vi "Process Memory Monitor.vi"() -> ()   [LabVIEW 2016]
panel:
  in  "Process Info Tab":enum32{"Page 1", "Page 2"}(tab)
  out "LabVIEW HandleCount":u32
  out "LabVIEW Thread Count":u32
  out "LabVIEW Memory Used (MB)":u64
  out "Sequence Editor Memory (MB)":u64
  out "Sequence Editor  HandleCount":u32
  out "Sequence Editor Thread Count":u32
  out "Process Memory Used (MB)":u64
  out "Process Thread Count":u32
  out "Process HandleCount":u32
  in  "Process Name (optional)":string
  in  "Log File Path":path=path "C:/Users/zhyang/Desktop/log.csv"
  in  "Interval (s)":dbl=3.0
  out "Memory Usage":cluster{"HandleCount":dbl, "HandleCount":dbl}(graph)
  out "error out":errorcluster
  in  "stop":bool
  # "Process Name is optional. If you let the control empty, this VI will monitor the LabVIEW and TestStand memory usage."
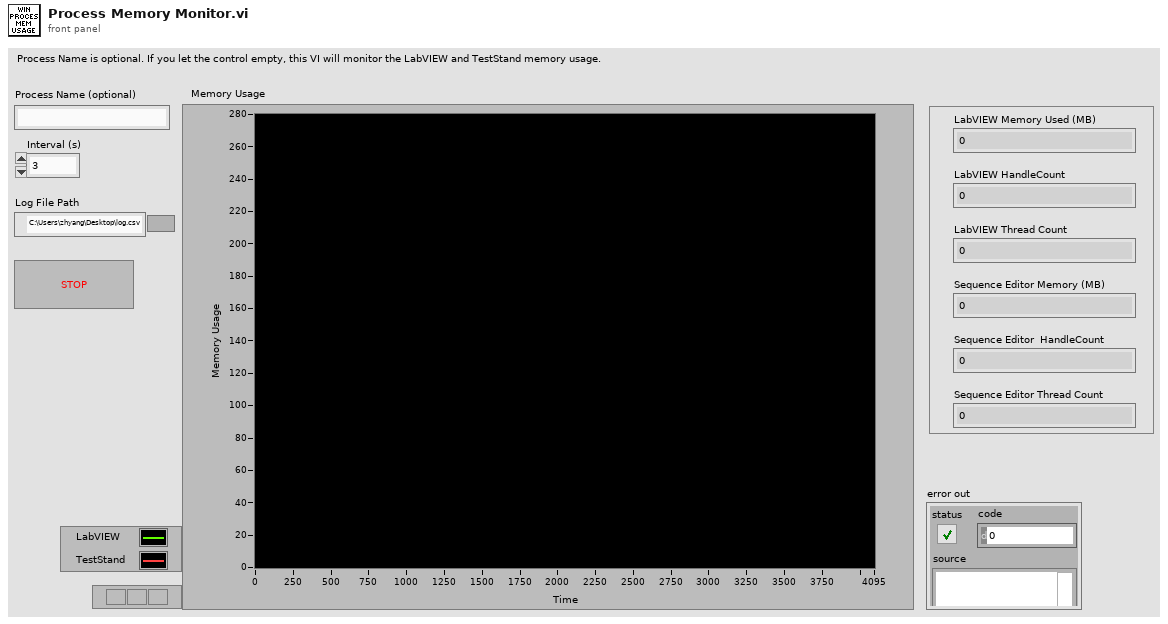
[diagram p1: front panel]
types:
  T1 = cluster{"LabVIEW  Memory Used (MB)":dbl, "Sequence Editor Memory (MB)":dbl}
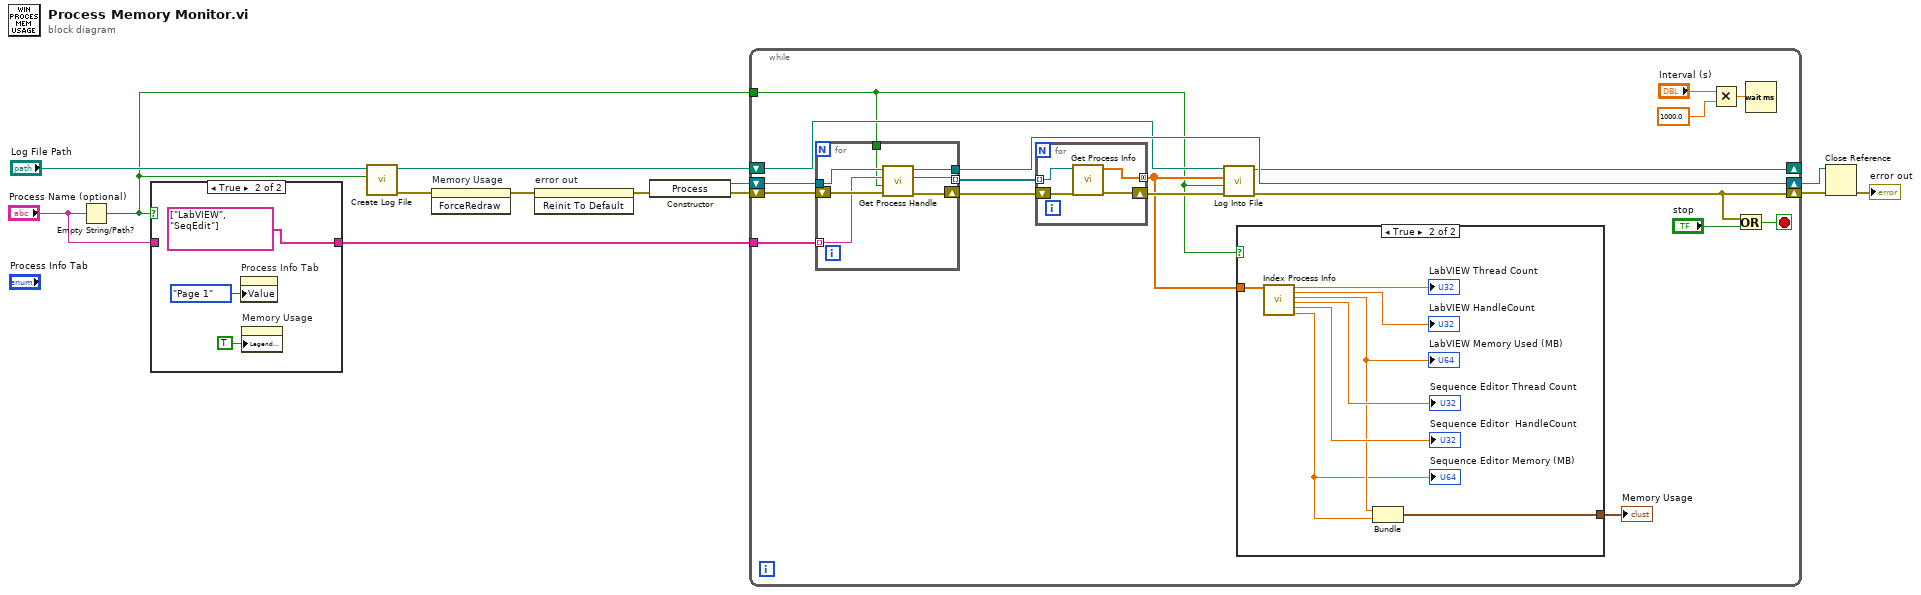
[diagram p0: block diagram]
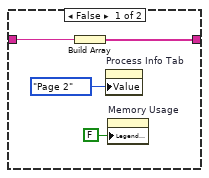
[diagram p2: hidden frame]
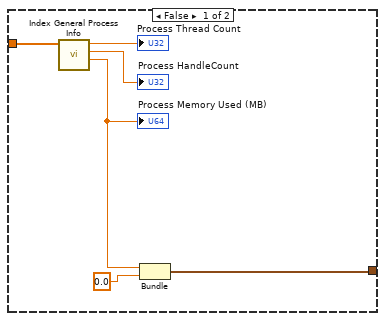
[diagram p3: hidden frame]
diagram:
  n1 = Empty String/Path?(string/path="Process Name (optional)") -> (empty?=w1:bool)
  n2 = case shown="True" w1 {
    tunnel: [w16 string[] ["LabVIEW", "SeqEdit"]] -> w2
    tunnel: "Process Name (optional)" -> [w17 _]
    frame False {
      n3 = Build Array(w17) -> (w16:string[])
      n4 = property on="Process Info Tab" class="TabCtl (strict)"("Value"=enum32{"Page 1", "Page 2"}."Page 2" ("Process Info Tab")) -> ()  [unwired: 2 in, 2 out]
      n5 = property on="Memory Usage" class="WFChart (strict)"("Legend Visible"=FALSE ("Legend:Visible")) -> ()  [unwired: 2 in, 2 out]
    }
    frame True {
      n6 = property on="Process Info Tab" class="TabCtl (strict)"("Value"=enum32{"Page 1", "Page 2"}."Page 1" ("Process Info Tab")) -> ()  [unwired: 2 in, 2 out]
      n7 = property on="Memory Usage" class="WFChart (strict)"("Legend Visible"=TRUE ("Legend:Visible")) -> ()  [unwired: 2 in, 2 out]
    }
  }
  n8 = call "Create Log File.vi"("Default Process?"=w1, "File Path (use dialog)"="Log File Path") -> ("error out"=w8:errorcluster, "log file path"=w7:path)  [unwired: 8 in]
  n9 = invoke on="Memory Usage" class="WFChart (strict)" method="ForceRedraw"(error in=w8) -> (error out=w5:errorcluster)  [unwired: 2 in, 2 out]
  n10 = invoke on="error out" class="Clust (strict)" method="Reinit To Default"(error in=w5) -> (error out=w4:errorcluster)  [unwired: 2 in, 2 out]
  n11 = constructor class="Process"(error in=w4) -> (reference out=w12:refnum<k24>, error out=w13:errorcluster)  [unwired: 2 in, 1 out]
  n12 = while {
    tunnel: w2 -> [w33]
    shift-right: [w24] -> w11
    shift-left: w13 -> [w34]
    shift-right: [w26] -> _
    shift-left: w7 -> [w27]
    shift-right: [w29] -> w10
    shift-left: w12 -> [w32]
    tunnel: w1 -> [w21]
    stop <- w25 stop-if-true
    n13 = for {
      tunnel: w33 -> [w60] mode=indexing
      tunnel: [w62] -> w29
      tunnel: w32 -> [w61]
      tunnel: [w59] -> w31 mode=indexing
      shift-right: [w58] -> w30
      shift-left: w34 -> [w63]
      tunnel: w21 -> [w57]
      n14 = call "Get Process Handle.vi"("error in (no error)"=w63, "Default Process?"=w57, "processName"=w60, ".NET Refnum in"=w61) -> ("error out"=w58:errorcluster, "target process handle"=w59:refnum<k24>, ".NET Refnum out"=w62:refnum<k24>)  [unwired: 5 in]
    }
    n15 = for {
      tunnel: w31 -> [w56] mode=indexing
      shift-right: [w54] -> w28
      shift-left: w30 -> [w55]
      tunnel: [w53] -> w22 mode=concatenating
      n16 = call "Get Process Info.vi"("error in (no error)"=w55, "process handle"=w56) -> ("error out"=w54:errorcluster, "process information"=w53:dbl[])  [unwired: 8 in]
    }
    n17 = call "Log Into File.vi"("error in"=w28, "Default Process?"=w21, "Memory Information"=w22, "file path in"=w27) -> ("error out"=w24:errorcluster, "file path out"=w26:path)  [unwired: 6 in]
    n18 = case shown="True" w21 {
      tunnel: [w41 w46] -> w23
      tunnel: w22 -> [w44 w45]
      frame False {
        n19 = call "Index General Process Info.vi"("process information"=w44) -> ("Process Memory Used (MB)"=w40:dbl, "Process HandleCount"=→"Process HandleCount":dbl, "Process Thread Count"=→"Process Thread Count":dbl)  [unwired: 8 in]
        "Process Memory Used (MB)" <- w40
        n20 = Bundle("Process Memory Used (MB)"=w40, 0.0) -> (w41:cluster{"Process Memory Used (MB)":dbl, dbl})  [unwired: 1 in]
      }
      frame True {
        n21 = call "Index Process Info.vi"("process information"=w45) -> ("LabVIEW Thread Count"=→"LabVIEW Thread Count":dbl, "LabVIEW HandleCount"=→"LabVIEW HandleCount":dbl, "LabVIEW  Memory Used (MB)"=w48:dbl, "Sequence Editor Thread Count"=→"Sequence Editor Thread Count":dbl, "Sequence Editor  HandleCount"=→"Sequence Editor  HandleCount":dbl, "Sequence Editor Memory (MB)"=w47:dbl)  [unwired: 13 in]
        "LabVIEW Memory Used (MB)" <- w48
        "Sequence Editor Memory (MB)" <- w47
        n22 = Bundle("LabVIEW  Memory Used (MB)"=w48, "Sequence Editor Memory (MB)"=w47) -> (w46:T1)  [unwired: 1 in]
      }
    }
    "Memory Usage" <- w23
    n23 = Multiply(x="Interval (s)", y=1000.0) -> (x*y=w37:dbl)
    n24 = Or(x=w24, y="stop") -> (x .or. y?=w25:bool)
    n25 = Wait (ms)(milliseconds to wait=w37) -> ()  [unwired: 1 out]
  }
  n26 = Close Reference(reference=w10, error in (no error)=w11) -> (error out=→"error out":errorcluster)
